vi "SlackAPI-auth.test.vi"(0 "token":string, 11 "error in (no error)":errorcluster) -> (4 "token out":string, 15 "error out":errorcluster)   [LabVIEW 2020]
uses:
  <vilib>/httpClient/POSTBuffer.vi
  <vilib>/httpClient/LabVIEWHTTPClient.lvlib
panel:
  out "body":string
  out "headers":string
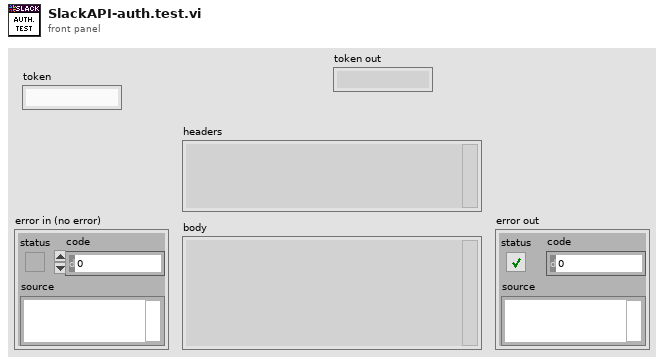
[diagram p1: front panel]
types:
  T1 = typedef "LabVIEWHTTPClient.lvlib/ClientHandle.ctl" = refnum<k1>
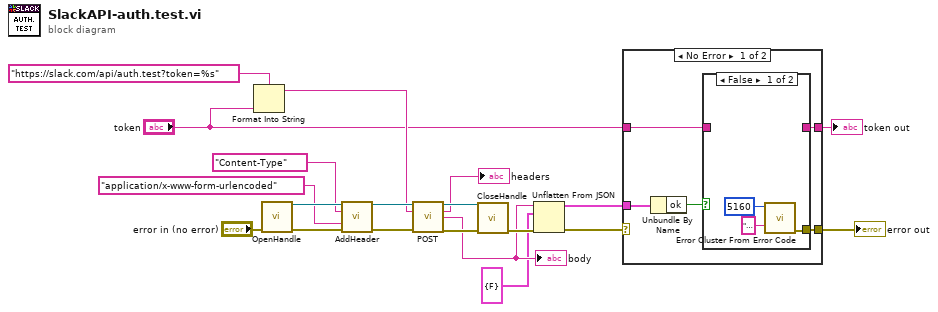
[diagram p0: block diagram]
diagram:
  n1 = Format Into String(format string="https://slack.com/api/auth.test?token=%s", "token") -> (resulting string=w13:string)  [unwired: 2 in, 1 out]
  n2 = call <vilib>:"OpenHandle.vi"("error in (no error)"="error in (no error)") -> ("client handle out"=w19:T1, "error out"=w20:errorcluster)  [unwired: 13 in]
  n3 = call <vilib>:"AddHeader.vi"("client handle"=w19, "header"="Content-Type", "value"="application/x-www-form-urlencoded", "error in (no error)"=w20) -> ("client handle out"=w15:T1, "error out"=w16:errorcluster)  [unwired: 10 in]
  n4 = call-poly <vilib>:"POST.vi"("client handle"=w15, "url"=w13, "error in (no error)"=w16) -> ("client handle out"=w12:T1, "headers"=→"headers":string, "body"=w7:string, "error out"=w11:errorcluster)  [unwired: 9 in]
  "body" <- w7
  n5 = call <vilib>:"CloseHandle.vi"("client handle"=w12, "error in (no error)"=w11) -> ("error out"=w8:errorcluster)  [unwired: 13 in]
  n6 = Unflatten From JSON(JSON string=w7, type and defaults=cluster{"ok":bool} {"ok"=FALSE}, error in (no error)=w8) -> (value=w4:cluster{"ok":bool}, error out=w5:errorcluster)  [unwired: 4 in]
  n7 = case shown="No Error" w5 {
    selector: w5 -> [_ w31]
    tunnel: w4 -> [w25 _]
    tunnel: [w23 w31] -> w3
    tunnel: "token" -> [w22 w30]
    tunnel: [w21 w30] -> w1
    frame No Error {
      n8 = Unbundle By Name(w25) -> ("ok"=w24:bool)
      n9 = case shown="False" w24 {
        tunnel: [w28 _] -> w23
        tunnel: w22 -> [_ w29]
        tunnel: [_ w29] -> w21
        frame False {
          n10 = call <vilib>:"Error Cluster From Error Code.vi"("error message (\"\")"="Failed Slack authorization test." ("error message (\"\")"), "error code (0)"=5160) -> ("error out"=w28:errorcluster)  [unwired: 7 in]
        }
        frame True {
        }
      }
    }
    frame Error {
    }
  }
  "error out" <- w3
  "token out" <- w1
